vi "Decode Fit Parameter Names & Values.vi"(8 "Error In":errorcluster, 11 "Fit Parameters":variant) -> (0 "Error Out":errorcluster, 1 "Parameter Values":dbl[](array[numeric]), 3 "Parameter Names":string[](array[string]))   [LabVIEW 2019]
uses:
  <vilib>/Utility/Data Type/NI_Data Type.lvlib
  Variant to Data.lvlib
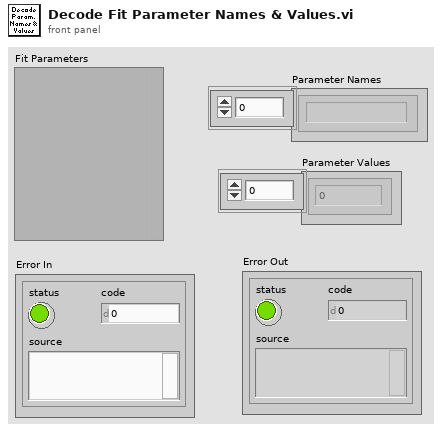
[diagram p1: front panel]
types:
  T1 = typedef "NI_Data Type.lvlib/Data Type.ctl" = enum8{"Invalid Type", "Void", "I8", "I16", "I32", "I64", "U8", "U16", "U32", "U64", "Single Float", "Double Float", "Extended Float", "Single Complex", "Double Complex", "Extended Complex", "Enum U8", "Enum U16", "Enum U32", "Enum U64", "Single Float With Unit", "Double Float With Unit", "Extended Float With Unit", "Single Complex with Unit", "Double Complex with Unit", "Extended Complex with Unit", "Boolean", "String", "Path", "Picture", "Tag", "Array", "Cluster", "Variant", "LV Variant", "Waveform", "Timestamp", "Digital Waveform", "Digital Data", "ExpressData", "Refnum", "External Data", "VI", "Poly VI", "LabVIEW Class Instance", "Fixed Point", "Set Collection", "Map Collection"}
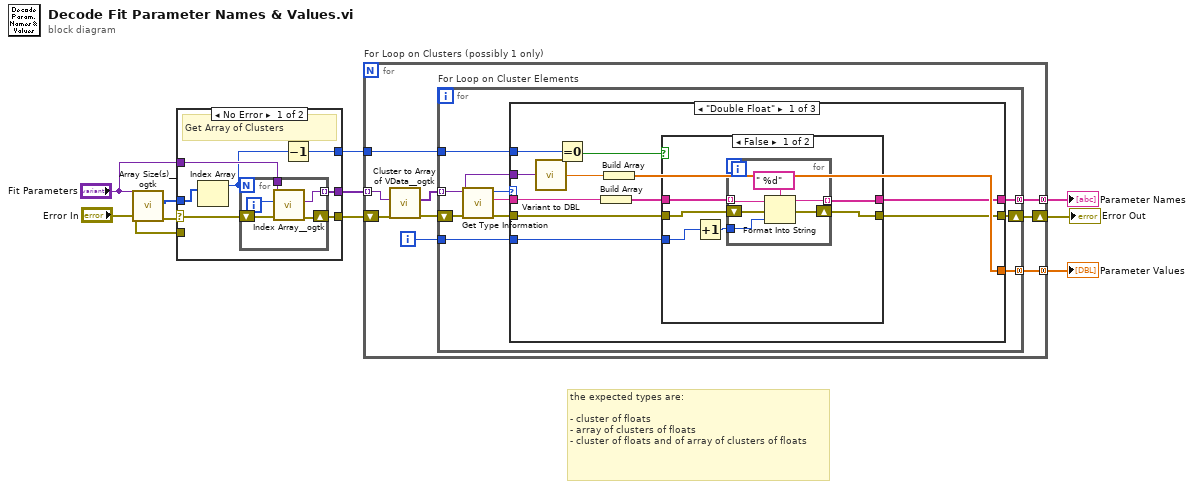
[diagram p0: block diagram]
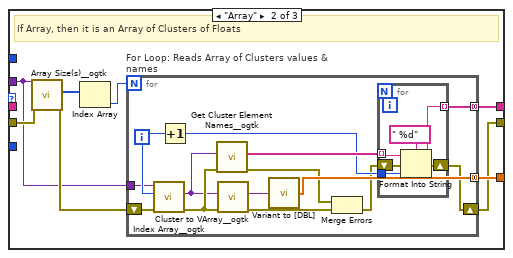
[diagram p3: hidden frame]
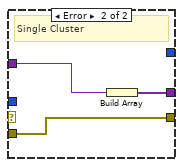
[diagram p5: hidden frame]
diagram:
  # "the expected types are:\n\n- cluster of floats\n- array of clusters of floats\n- cluster of floats and of array of clusters of floats"
  n1 = call <userlib>:"Array Size(s)__ogtk.vi"("error in (no error)"="Error In", "Array"="Fit Parameters") -> ("error out"=w3:errorcluster, "Size(s)"=w2:u32[])  [unwired: 7 in, 1 out]
  n2 = case shown="No Error" w3 {
    selector: w3 -> [w16 _]
    tunnel: "Fit Parameters" -> [w17 w24]
    tunnel: [w15 w25] -> w7
    tunnel: [w14 w23] -> w6
    tunnel: "Error In" -> [_ w25]
    tunnel: w2 -> [w13 _]
    tunnel: [w11 _] -> w1
    frame No Error {
      # "Get Array of Clusters"
      n3 = Index Array(array=w13) -> (element=w12:u32)  [unwired: 1 in]
      n4 = for {
        N: w12 -> [_]
        tunnel: w17 -> [w21]
        tunnel: [w20] -> w14 mode=indexing
        shift-right: [w18] -> w15
        shift-left: w16 -> [w19]
        i -> [w22]
        n5 = call <userlib>:"Index Array__ogtk.vi"("error in (no error)"=w19, "Index (1D)"=w22, "MultiD Array"=w21) -> ("error out"=w18:errorcluster, "Array Element"=w20:variant)  [unwired: 7 in]
      }
      n6 = Decrement(x=w12) -> (x-1=w11:u32)
    }
    frame Error {
      # "Single Cluster"
      n7 = Build Array(w24) -> (w23:variant[])
    }
  }
  n8 = for "For Loop on Clusters (possibly 1 only)" {
    tunnel: [w32] -> w10 mode=concatenating
    tunnel: [w31] -> w9 mode=concatenating
    shift-right: [w30] -> w8
    shift-left: w7 -> [w29]
    tunnel: w6 -> [w28] mode=indexing
    tunnel: w1 -> [w27]
    i -> [w26]
    n9 = call <userlib>:"Cluster to Array of VData__ogtk.vi"("error in (no error)"=w29, "Cluster"=w28) -> ("error out"=w34:errorcluster, "Array of VData"=w33:variant[])  [unwired: 8 in]
    n10 = for "For Loop on Cluster Elements" {
      tunnel: w33 -> [w40] mode=indexing
      shift-right: [w38] -> w30
      shift-left: w34 -> [w44]
      tunnel: [w41] -> w32 mode=concatenating
      tunnel: [w39] -> w31 mode=concatenating
      tunnel: w27 -> [w36]
      tunnel: w26 -> [w35]
      n11 = call <vilib>:"Get Type Information.vi"("error in (no error)"=w44, "variant"=w40) -> ("error out"=w42:errorcluster, "name"=w37:string, "type"=w43:T1)  [unwired: 5 in, 2 out]
      n12 = case shown="\"Double Float\"" w43 {
        tunnel: w37 -> [w55 _ _]
        tunnel: w42 -> [w46 w77 w98]
        tunnel: [w48 w74 _] -> w41
        tunnel: w40 -> [w54 w71 _]
        tunnel: [w52 w73 _] -> w39
        tunnel: [w45 w72 w98] -> w38
        tunnel: w36 -> [w51 _ _]
        tunnel: w35 -> [w47 _ _]
        frame "Double Float" {
          n13 = call "Variant to DBL.vi"("Variant"=w54) -> ("Value"=w53:dbl)  [unwired: 8 in]
          n14 = Equal To 0?(x=w51) -> (x = 0?=w50:bool)
          n15 = Build Array(w55) -> (w49:string[])
          n16 = Build Array(w53) -> (w52:dbl[])
          n17 = case shown="False" w50 {
            tunnel: w49 -> [w61 w69]
            tunnel: [w60 w69] -> w48
            tunnel: w47 -> [w59 _]
            tunnel: w46 -> [w57 w68]
            tunnel: [w56 w68] -> w45
            frame False {
              n18 = Increment(x=w59) -> (x+1=w58:i32)
              n19 = for {
                tunnel: w61 -> [w67] mode=indexing
                tunnel: [w65] -> w60 mode=indexing
                tunnel: w58 -> [w64]
                shift-right: [w62] -> w56
                shift-left: w57 -> [w63]
                n20 = Format Into String(format string=" %d", initial string=w67, error in=w63, w64) -> (resulting string=w65:string, error out=w62:errorcluster)
              }
            }
            frame True {
            }
          }
        }
        frame "Array" {
          # "If Array, then it is an Array of Clusters of Floats"
          n21 = call <userlib>:"Array Size(s)__ogtk.vi"("error in (no error)"=w77, "Array"=w71) -> ("error out"=w75:errorcluster, "Size(s)"=w76:u32[])  [unwired: 7 in, 1 out]
          n22 = Index Array(array=w76) -> (element=w70:u32)  [unwired: 1 in]
          n23 = for "For Loop: Reads Array of Clusters values & names" {
            N: w70 -> [_]
            shift-right: [w78] -> w72
            shift-left: w75 -> [w91]
            tunnel: [w85] -> w74 mode=concatenating
            tunnel: [w83] -> w73 mode=concatenating
            tunnel: w71 -> [w81]
            i -> [w87]
            n24 = call <userlib>:"Index Array__ogtk.vi"("error in (no error)"=w91, "Index (1D)"=w87, "MultiD Array"=w81) -> ("error out"=w89:errorcluster, "Array Element"=w88:variant)  [unwired: 7 in]
            n25 = Increment(x=w87) -> (x+1=w80:i32)
            n26 = call <userlib>:"Get Cluster Element Names__ogtk.vi"("error in (no error)"=w89, "Cluster"=w88) -> ("error out"=w82:errorcluster, "Element Names"=w86:string[])  [unwired: 8 in]
            n27 = call <userlib>:"Cluster to VArray__ogtk.vi"("error in (no error)"=w89, "Cluster"=w88) -> ("error out"=w90:errorcluster, "VArray"=w84:variant)  [unwired: 8 in]
            n28 = call "Variant to [DBL].vi"("Variant"=w84) -> ("Value"=w83:dbl[])  [unwired: 8 in]
            n29 = Merge Errors(w82, w90) -> (w79:errorcluster)
            n30 = for {
              tunnel: w86 -> [w97] mode=indexing
              tunnel: [w95] -> w85 mode=indexing
              tunnel: w80 -> [w94]
              shift-right: [w92] -> w78
              shift-left: w79 -> [w93]
              n31 = Format Into String(format string=" %d", initial string=w97, error in=w93, w94) -> (resulting string=w95:string, error out=w92:errorcluster)
            }
          }
        }
        frame "Cluster", Default {
          # "unknown type"
        }
      }
    }
  }
  "Parameter Names" <- w10
  "Parameter Values" <- w9
  "Error Out" <- w8
